vi "decodeClusterRef.vi"(8 "error in (no error)":errorcluster, 10 "Cluster Reference":refnum<vi>, 11 "variant":variant) -> (0 "error out":errorcluster)   [LabVIEW 2015, in "MsgPack.lvlib"]
uses:
  MsgPack.lvlib
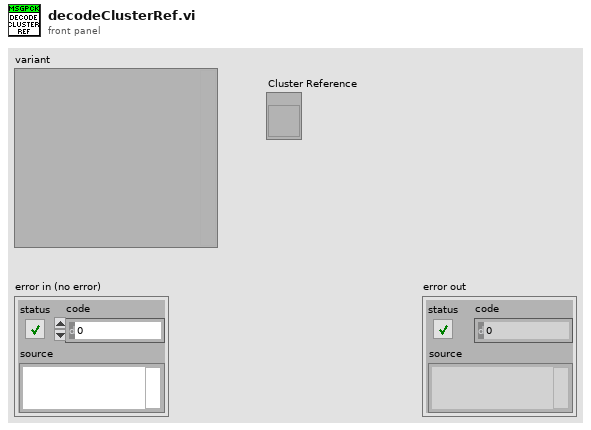
[diagram p1: front panel]
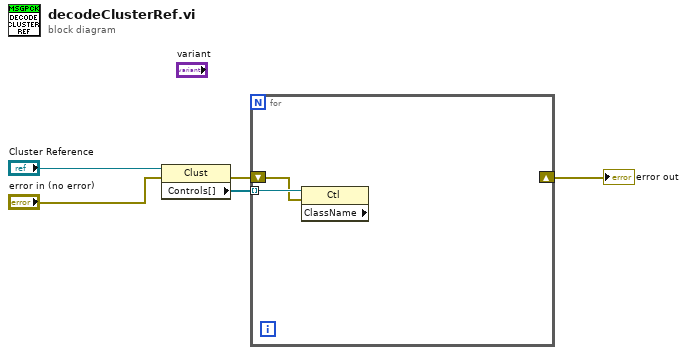
[diagram p0: block diagram]
diagram:
  n1 = property class="Clust"(reference="Cluster Reference", error in="error in (no error)") -> (error out=w2:errorcluster, "Controls[]"=w3:refnum<vi>[])  [unwired: 1 out]
  n2 = for {
    tunnel: w3 -> [w7] mode=indexing
    shift-right: [_] -> w1
    shift-left: w2 -> [w6]
    n3 = property class="Ctl" props=["ClassName"](reference=w7, error in=w6) -> ()  [unwired: 3 out]
  }
  "error out" <- w1
